vi "test_TCP_2_ convert_Number_to_packet.vi"(11 "input_Number":i32) -> (2 "output_PrePacket":string, 3 "output_packet":string)   [LabVIEW 2014]
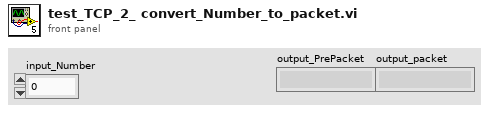
[diagram p1: front panel]
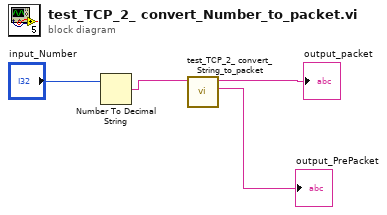
[diagram p0: block diagram]
diagram:
  n1 = Number To Decimal String(number="input_Number") -> (decimal integer string=w3:string)  [unwired: 1 in]
  n2 = call "test_TCP_2_ convert_String_to_packet.vi"("input_string"=w3) -> ("output_PrePacket"=→"output_PrePacket":string, "output_packet"=→"output_packet":string)  [unwired: 9 in]
